vi "From Bool Tree Data.vi"(11 "Tree Data":refnum<class "Tree Data.lvclass">) -> (2 "Boolean":bool)   [LabVIEW 2020, in "NI_VIAnCFGDataStructure.lvlib" / "Bool.lvclass"]
doc: "Extract a Bool value from Tree Data type."
uses:
  <vilib>/addons/analyzer/VIAnCFGDataStructure/Data Types/Bool/Bool.lvclass
  <vilib>/addons/analyzer/VIAnCFGDataStructure/Tree Data/Tree Data.lvclass
  <vilib>/addons/analyzer/VIAnCFGDataStructure/Data Types/Bool/Bool.lvclass/Bool.ctl
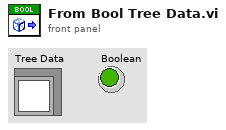
[diagram p1: front panel]
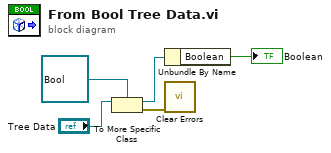
[diagram p0: block diagram]
diagram:
  n1 = To More Specific Class(target class=refnum<class "Bool.lvclass"> refnum ("Tree Data"), reference="Tree Data") -> (specific class reference=w2:refnum<class "Bool.lvclass">, error out=w1:errorcluster)  [unwired: 1 in]
  n2 = Unbundle By Name(w2) -> ("Boolean"=→"Boolean":bool)
  n3 = call <vilib>:"Clear Errors.vi"("error in (no error)"=w1) -> ()  [unwired: 5 in, 2 out]
